vi "Remove Multiple Custom Device Items by Path.vi"(8 "error in":errorcluster, 10 "Paths of Items to Remove":string[](array[string]), 11 "Device Item Ref in":T1 format="%.0x") -> (0 "error out":errorcluster, 3 "Device Item Ref out":T1 format="%.0x")   [LabVIEW 2020, in "Vires VTD System Explorer.lvlib"]
uses:
  Vires VTD System Explorer.lvlib
  <vilib>/NI VeriStand/Custom Device API/Custom Device Item Ref.ctl
  <vilib>/NI VeriStand/Custom Device API/Custom Device API.lvlib
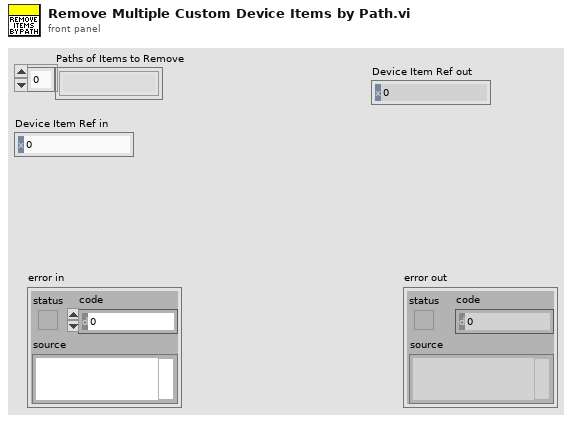
[diagram p1: front panel]
types:
  T1 = typedef "Custom Device API.lvlib/Custom Device Item Ref.ctl" = u64
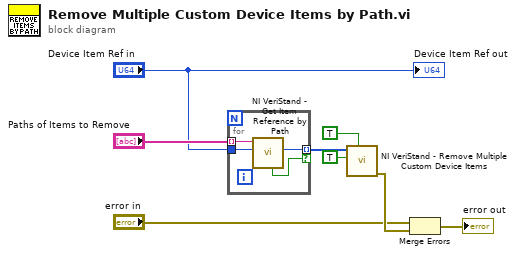
[diagram p0: block diagram]
diagram:
  n1 = for {
    tunnel: "Device Item Ref in" -> [w11]
    tunnel: "Paths of Items to Remove" -> [w12] mode=indexing
    tunnel: [w10] -> w6 mode=indexing if=w9
    n2 = call <vilib>:"NI VeriStand - Get Item Reference by Path.vi"("Root Ref"=w11, "Item Path in"=w12) -> ("Item Ref"=w10:T1, "Found"=w9:bool)  [unwired: 6 in, 2 out]
  }
  n3 = call <vilib>:"NI VeriStand - Remove Multiple Custom Device Items.vi"("Skip action VI on delete (F)"=TRUE, "Force Delete (F)"=TRUE, "Item Refs in"=w6) -> ("error out"=w3:errorcluster)  [unwired: 7 in, 1 out]
  n4 = Merge Errors("error in", w3) -> (→"error out":errorcluster)
  "Device Item Ref out" <- "Device Item Ref in"
